vi "Host.vi"() -> ()   [LabVIEW 2025]
uses:
  <vilib>/Handler Framework/CmdQueue/Enqueue Single.vi
  Classes/Processor/Processor.lvclass
  <vilib>/Handler Framework/Handler Framework.lvlib
panel:
  out "error out":errorcluster
  in  "Measure":bool
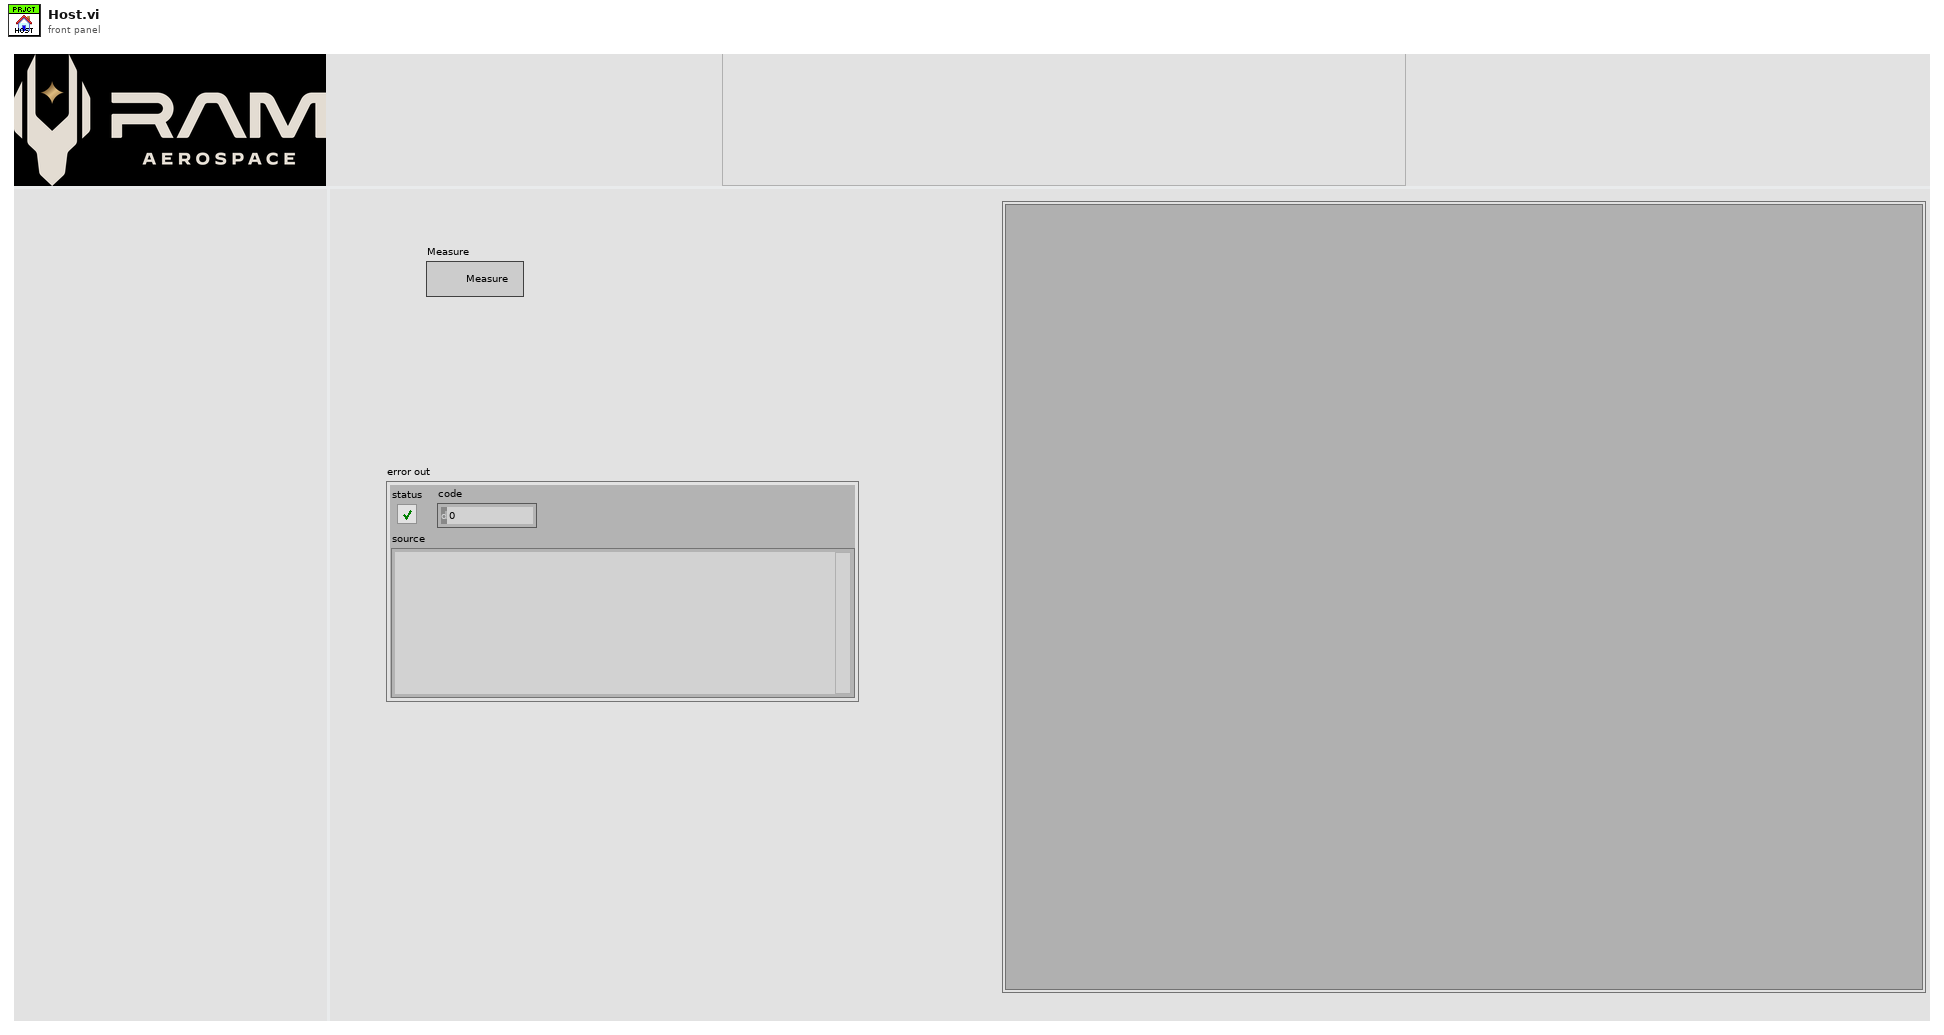
[diagram p1: front panel]
types:
  T1 = cluster{"Thermal Tape":refnum<class "Processor.lvclass">, "Thermocouples":refnum<class "Processor.lvclass">}
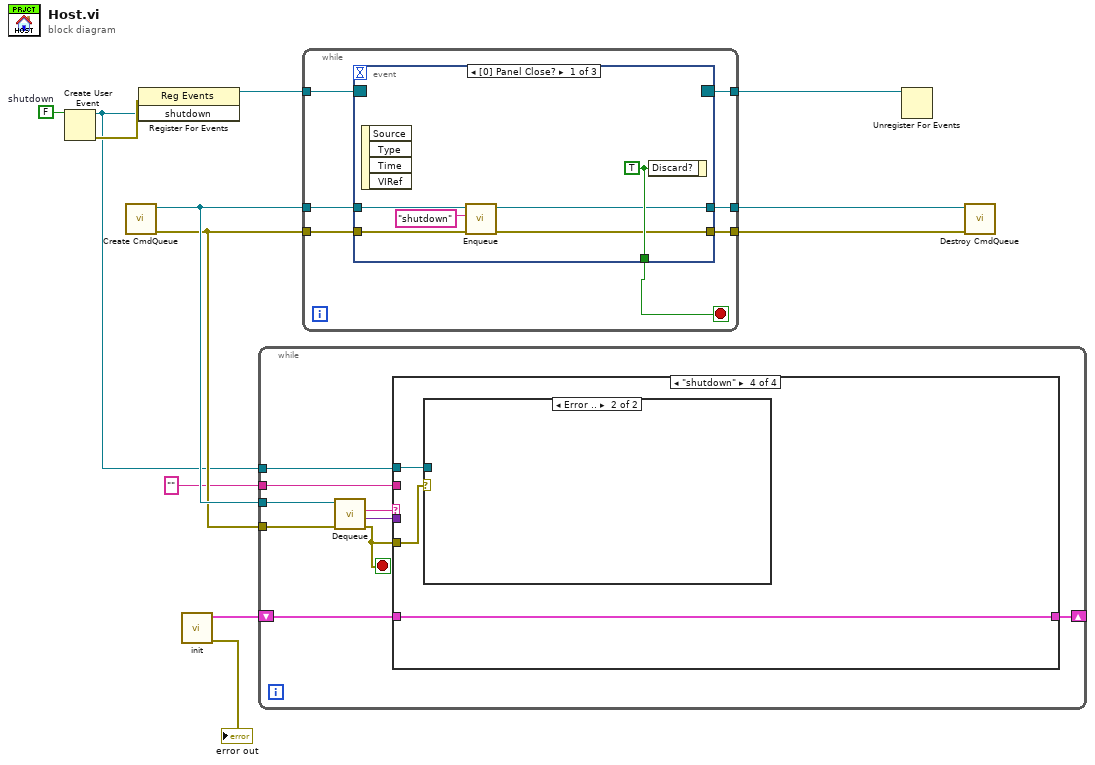
[diagram p0: block diagram]
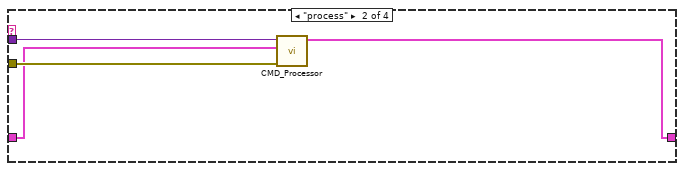
[diagram p3: hidden frame]
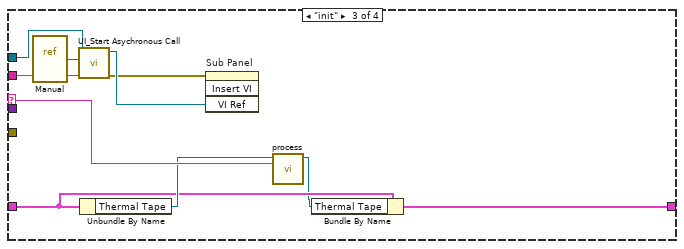
[diagram p4: hidden frame]
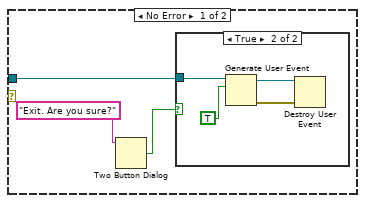
[diagram p5: hidden frame]
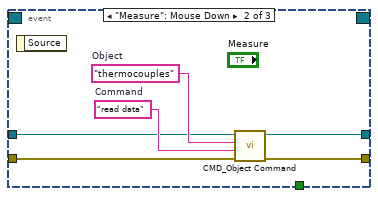
[diagram p7: hidden frame]
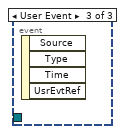
[diagram p8: hidden frame]
diagram:
  w8 = FALSE  # shutdown
  n1 = Create User Event(user event datatype=w8) -> (user event=w3:refnum<user-event>, error out=w4:errorcluster)  [unwired: 1 in]
  n2 = call <vilib>:"Create CmdQueue.vi"() -> ("error out"=w9:errorcluster, "CmdQueue out"=w10:refnum<queue>)  [unwired: 10 in]
  n3 = register-events(error in=w4, w3) -> (reference out=w7:refnum<event-registration>)  [unwired: 1 in, 1 out]
  n4 = call "init.vi"() -> ("error out"=→"error out":errorcluster, "objects"=w2:T1)  [unwired: 10 in]
  n5 = while {
    tunnel: w10 -> [w21]
    tunnel: w9 -> [w18]
    tunnel: w3 -> [w17]
    tunnel: "" ("String") -> [w16]
    shift-right: [w13] -> _
    shift-left: w2 -> [w14]
    stop <- w15 stop-if-true
    n6 = call <vilib>:"Dequeue.vi"("error in (no error)"=w18, "CmdQueue in"=w21) -> ("error out"=w15:errorcluster, "value"=w19:variant, "cmd"=w20:string)  [unwired: 5 in, 2 out]
    n7 = case shown="\"shutdown\"" w20 {
      selector: w20 -> [_ _ w31 _]
      tunnel: w19 -> [_ w26 _ _]
      tunnel: w17 -> [_ _ w33 w39]
      tunnel: w16 -> [_ _ w32 _]
      tunnel: w15 -> [_ w25 _ w38]
      tunnel: w14 -> [w22 w24 w29 w37]
      tunnel: [w22 w23 w27 w37] -> w13
      frame "False", Default {
      }
      frame "process" {
        n8 = call "CMD_Processor.vi"("error in (no error)"=w25, "objects in"=w24, "Object + CMD"=w26) -> ("objects out"=w23:T1)  [unwired: 6 in, 2 out]
      }
      frame "init" {
        n9 = vi-ref "Manual.vi"() -> (w36:refnum<vi>)
        n10 = call "UI_Start Asychronous Call.vi"("String"=w32, "VI Refnum"=w36, "User Event in"=w33) -> ("error out"=w34:errorcluster, "VI out"=w35:refnum<vi>)  [unwired: 7 in]
        n11 = Unbundle By Name(w29) -> ("Thermal Tape"=w30:refnum<class "Processor.lvclass">)
        n12 = invoke on="Sub Panel" class="SubPnl" method="Insert VI"(error in=w34, "VI Ref"=w35) -> ()  [unwired: 2 in, 4 out]
        n13 = call-dynamic "process.vi"("Process"=w31, "Processor in"=w30) -> ("Processor out"=w28:refnum<class "Processor.lvclass">)  [unwired: 7 in, 2 out]
        n14 = Bundle By Name(cluster=w29, "Thermal Tape"=w28) -> (w27:T1)
      }
      frame "shutdown" {
        n15 = case shown="Error .." w38 {
          tunnel: w39 -> [w40 _]
          frame No Error {
            n16 = Two Button Dialog(message="Exit. Are you sure?") -> (T button?=w41:bool)  [unwired: 2 in]
            n17 = case shown="True" w41 {
              tunnel: w40 -> [_ w46]
              frame False {
              }
              frame True {
                n18 = Generate User Event(user event=w46, event data cluster=TRUE ("event data")) -> (user event out=w44:refnum<user-event>, error out=w43:errorcluster)  [unwired: 2 in]
                n19 = Destroy User Event(user event=w44, error in=w43) -> ()  [unwired: 1 out]
              }
            }
          }
          frame Error {
          }
        }
      }
    }
  }
  n20 = while {
    tunnel: w10 -> [w51]
    tunnel: [w49] -> w12
    tunnel: w9 -> [w50]
    tunnel: [w48] -> w11
    tunnel: w7 -> [w53]
    tunnel: [w52] -> w6
    stop <- w47 stop-if-true
    n21 = event shown="[0] Panel Close?" {
      selector: w53 -> [_ _ _]
      dyn-events: [_ _ _] -> w52
      timeout: _ -> [_ _ _]
      tunnel: w51 -> [w58 w61 _]
      tunnel: w50 -> [w57 w60 _]
      tunnel: [w55 w65 _] -> w49
      tunnel: [w54 _ _] -> w48
      tunnel: [w56 _ _] -> w47
      tunnel: [_ w64 _] -> _
      event Panel Close? {
        w56 = TRUE ("Discard?")
        n22 = event-data() -> ()  [unwired: 1 in, 4 out]
        n23 = call-poly <vilib>:"Enqueue.vi"("error in (no error)"=w57, "Command"="shutdown", "CmdQueue in"=w58) -> ("error out"=w54:errorcluster, "CmdQueue out"=w55:refnum<queue>)  [unwired: 7 in]
        n24 = event-data("Discard?"=w56) -> ()  [unwired: 1 in, 1 out]
      }
      event "Measure": Mouse Down {
        w62 = "read data"  # Command
        w63 = "thermocouples"  # Object
        n25 = event-data() -> ()  [unwired: 1 in, 1 out]
        n26 = call "CMD_Object Command.vi"("error in (no error)"=w60, "Command"=w62, "Object"=w63, "Queue in"=w61) -> ("error out"=w64:errorcluster, "Queue out"=w65:refnum<queue>)  [unwired: 6 in]
      }
      event User Event {
        n27 = event-data() -> ()  [unwired: 1 in, 4 out]
      }
    }
  }
  n28 = Unregister For Events(event registration refnum=w6) -> ()  [unwired: 1 in, 1 out]
  n29 = call <vilib>:"Destroy CmdQueue.vi"("error in (no error)"=w11, "CmdQueue in"=w12) -> ()  [unwired: 9 in, 1 out]
